vi "CPP_Aeroprobe-MultiProbeQuick.vi"() -> (5 "Plug in titles":string[](array[string]), 7 "Plug in values":string[](array[string]))   [LabVIEW 2013]
uses:
  Globals/Meas_global.vi
  Globals/Trav_pos_global.vi
panel:
  out "MultiProbeCals":string caption="DelimitedCalFileList (for MultiProbe)"
  in  "Calibration Folder Path":path=path "G:/5HoleProbe"
  in  "Old5HoleProbe?":bool
  in  "Mode":enum32{"Measure", "Take Zeroes"}(radio)=enum."Take Zeroes"
  in  "RunManually?":bool
  out "return type":i32
  out "p-p0":dbl[](array[numeric]) format="%#.5f"
  out "Temperature/C":dbl format="%#.1f"
  out "Pressure/mBar":dbl
  out "timeOfzero":timestamp
  out "zeroShift/mmH2O":dbl[](array[numeric]) format="%#.6f"
  out "Velocity":dbl
  out "W":dbl
  out "V":dbl
  out "U":dbl caption="u  m/s"
  # "!! 5-hole 1-5 must be connected to Channels 1-5 !!"
  # "Zero Info"
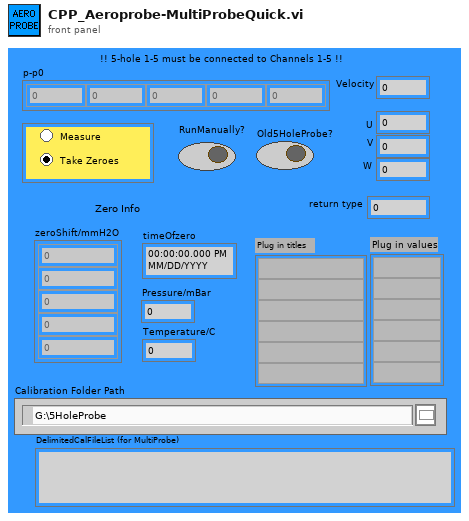
[diagram p1: front panel]
types:
  T1 = typedef "Post_Process.ctl" = enum16{"Take New Data", "Post Process Raw Data File"}
  T2 = typedef "Traverse_cluster.ctl" = cluster{"Start X":dbl, "Start Y":dbl, "Start Z":dbl, "End X":dbl, "End Y":dbl, "End Z":dbl, "No. of pts.":i32, "Spacing":T3, "Filename":path, "Tunnel Speed":dbl, "Averaging time (min)":dbl, "Extra Commands":string, "Specific Arguments":string, "Emission Rate (l/min)":dbl, "Trace Gas Concentration (%)":dbl, "Density Ratio":string, "Comments":string, "Row No":i32, "Row Type Selector":T4, "Completion time":string, "Row Duration (mins)":dbl, "No. of Valid pts.":i32, "Meas Setup File":string}
  T3 = typedef "Spacing.ctl" = enum16{"Linear", "Log", "Gauss", "Specified", "N/A"}
  T4 = typedef "Multi_run_mode.ctl" = enum16{"Move Traverse Only", "Set Tunnel Speed Only", "Set Source Only", "Set Measurement Conditions", "Single Measurement", "Vertical Profile", "Lateral Profile", "Longitudinal Profile", "Explore Volume", "Multi-Axis Profile", "Auto Calibrate", "Meas Fast FID Bkgnd", "Check Beam Power", "Scanning Valve Measurement", "Run VI Named:", "Set ADAM Ch", "Wait (minutes)", "Send Message", "Synchronize With:", "Fall Back to this Row", "Turn Off Row Repeating", "Blank Row", "Traverse 3D Volume"}
  T5 = typedef "Analysis_info_cluster.ctl" = cluster{"Colour":u32, "Inst type":T6, "Inst name":string, "Symbol":string, "Code name":string, "Extra Info":string, "Inst Array":T7, "Extra Titles":string[], "Extra Values":string[], "U":dbl, "u^2":dbl, "u^3":dbl, "u^4":dbl, "Skew_u":dbl, "Kurt_u":dbl, "Sd Error in Mean":dbl, "% u'/U":dbl, "X":dbl, "Y":dbl, "Z":dbl, "Timescale integral to 25%":dbl, "Sd Error in Variance":dbl, "Calib File":path, "Calib Constants":dbl[], "Output Position":bool, "Full Stats":bool, "Av Sampling Rate":dbl, "Av No of Samples":dbl, "Total Meas Time (s)":dbl, "ADAM Ch Name":string}
  T6 = typedef "Inst_type.ctl" = enum16{"Propeller anemometer", "Raw voltage", "Pressure Transducer", "Pitot-static tube", "Preston tube", "Hot wire", "Cross wire 1", "Cross wire 2", "Generic Linear", "Generic Polynomial", "Generic BackPoly", "Fast FID", "Thermocouple", "Cold wire", "Pulsed Wire", "LDA Vel", "LDA Tran time", "LDA Arr time"}
  T7 = typedef "Instrument_Array.ctl" = enum16{"PWA", "LDA", "Analogue"}
  T8 = cluster{"Analysis Info cluster[0]":T5, "Analysis Info cluster[1]":T5, "Analysis Info cluster[2]":T5, "Analysis Info cluster[3]":T5, "Analysis Info cluster[4]":T5, "Analysis Info cluster[5]":T5, "Analysis Info cluster[6]":T5}
  T9 = cluster{"Analysis Info cluster[0]":T5, "Analysis Info cluster[1]":T5, "Analysis Info cluster[2]":T5, "Analysis Info cluster[3]":T5, "Analysis Info cluster[4]":T5, "Analysis Info cluster[5]":T5, "Analysis Info cluster[6]":T5, "Analysis Info cluster[7]":T5, "Analysis Info cluster[8]":T5, "Analysis Info cluster[9]":T5, "Analysis Info cluster[10]":T5, "Analysis Info cluster[11]":T5, "Analysis Info cluster[12]":T5, "Analysis Info cluster[13]":T5}
  T10 = cluster{"[0]":dbl, "[1]":dbl, "[2]":dbl, "[3]":dbl, "[4]":dbl}
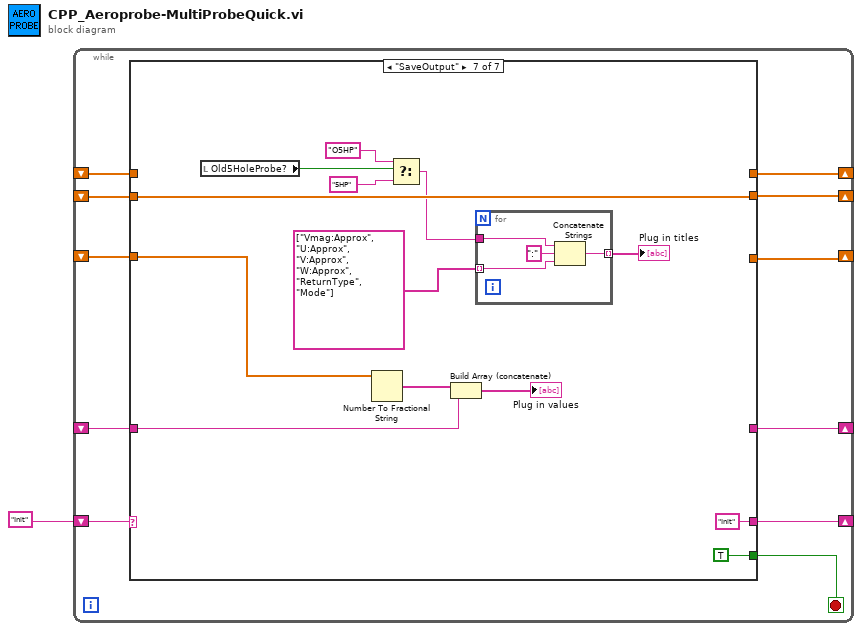
[diagram p0: block diagram]
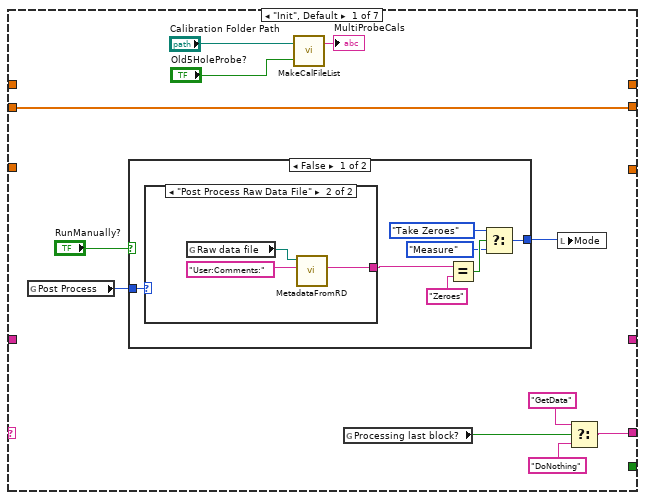
[diagram p2: hidden frame]
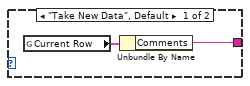
[diagram p3: hidden frame]
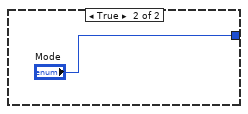
[diagram p4: hidden frame]
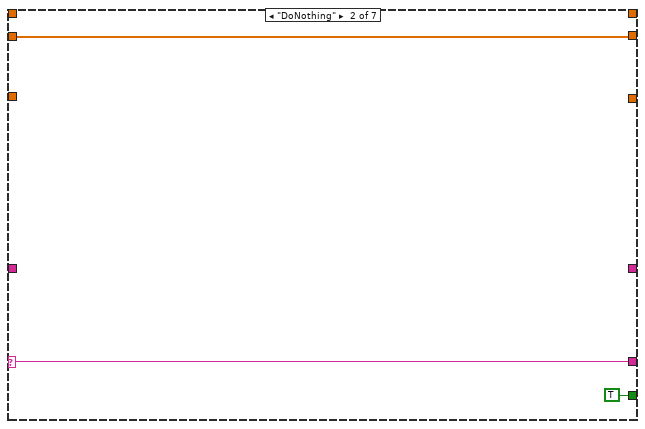
[diagram p5: hidden frame]
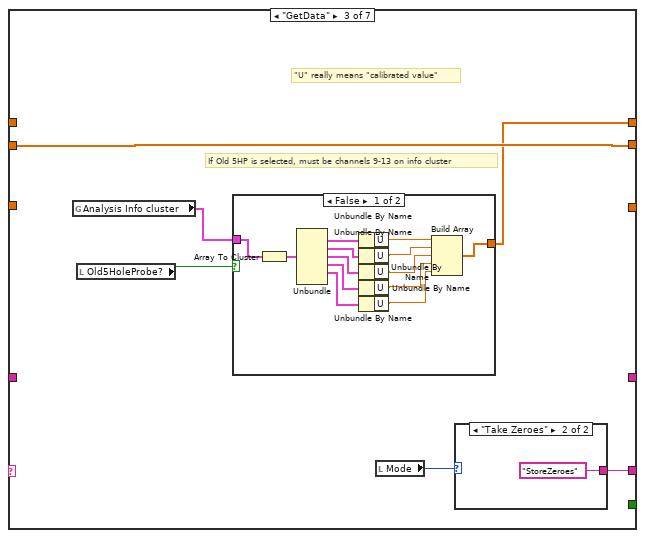
[diagram p6: hidden frame]
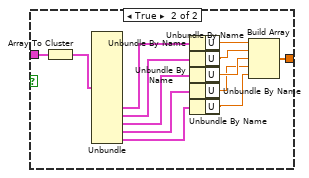
[diagram p7: hidden frame]
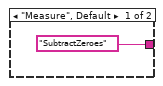
[diagram p8: hidden frame]
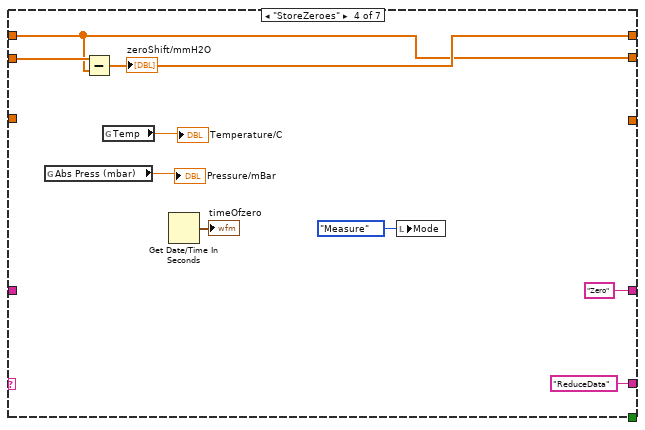
[diagram p9: hidden frame]
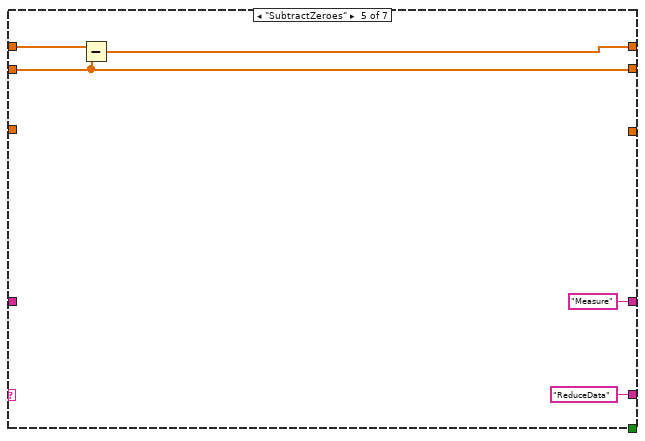
[diagram p10: hidden frame]
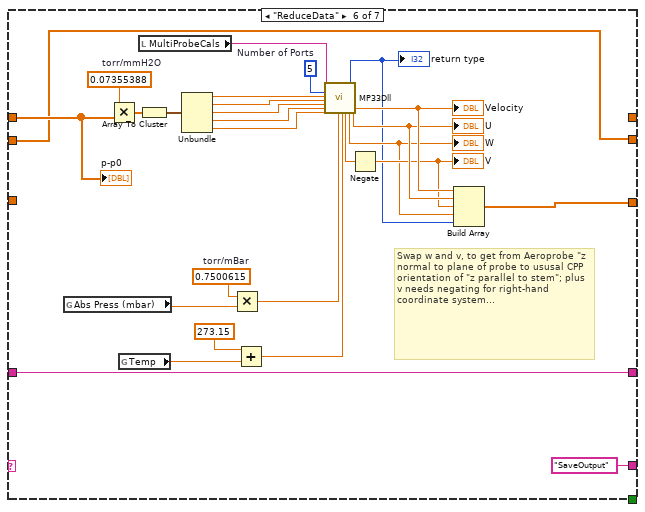
[diagram p11: hidden frame]
diagram:
  n1 = while {
    shift-right: [w11] -> _
    shift-left: "Init" -> [w12]
    shift-right: [w10] -> _
    shift-left: _ -> [w8]
    shift-right: [w9] -> _
    shift-left: _ -> [w7]
    shift-right: [w6] -> _
    shift-left: _ -> [w5]
    shift-right: [w3] -> _
    shift-left: _ -> [w2]
    stop <- w4 stop-if-true
    n2 = case shown="\"SaveOutput\"" w12 {
      selector: w12 -> [_ w39 _ _ _ _ _]
      tunnel: [w23 w39 w45 "ReduceData" "ReduceData" "SaveOutput" "Init"] -> w11
      tunnel: [_ _ w42 w80 w86 _ _] -> w10
      tunnel: [w19 w37 w44 w74 w85 w99 w127] -> w9
      tunnel: w8 -> [_ _ _ w74 w87 w108 _]
      tunnel: w7 -> [w19 w37 w44 w82 w85 w99 w127]
      tunnel: [_ _ _ _ _ w95 _] -> w6
      tunnel: w5 -> [_ _ _ _ _ _ w126]
      tunnel: [_ TRUE _ _ _ _ TRUE] -> w4
      tunnel: [_ _ _ "Zero" "Measure" w94 _] -> w3
      tunnel: w2 -> [_ _ _ _ _ w94 w121]
      frame "Init", Default {
        n3 = global read "Meas_global.vi" "Post Process"() -> (w16:T1)
        n4 = case shown="False" "RunManually?" {
          tunnel: [w30 "Mode"] -> w17
          tunnel: w16 -> [w24 _]
          frame False {
            n5 = case shown="\"Post Process Raw Data File\"" w24 {
              tunnel: [w31 w33] -> w29
              frame "Take New Data", Default {
                n6 = global read "Trav_pos_global.vi" "Current Row"() -> (w32:T2)
                n7 = Unbundle By Name(w32) -> ("Comments"=w31:string)
              }
              frame "Post Process Raw Data File" {
                n8 = global read "Meas_global.vi" "Raw data file"() -> (w35:path)
                n9 = call "MetadataFromRD.vi"("ChannelName"="User:Comments:", "Raw data file"=w35) -> ("ValueString"=w33:string)  [unwired: 8 in, 1 out]
              }
            }
            n10 = Equal?(x=w29, y="Zeroes") -> (x = y?=w27:bool)
            n11 = Select(t=enum32{"Measure", "Take Zeroes"}."Take Zeroes" ("Mode"), s=w27, f=enum32{"Measure", "Take Zeroes"}."Measure" ("Mode")) -> (s? t:f=w30:enum32{"Measure", "Take Zeroes"})
          }
          frame True {
          }
        }
        n12 = call "MakeCalFileList.vi"("Old5HoleProbe?"="Old5HoleProbe?", "Calibration Folder Path"="Calibration Folder Path") -> ("MultiProbeCals"=→"MultiProbeCals":string)  [unwired: 1 out]
        n13 = global read "Meas_global.vi" "Processing last block?"() -> (w22:bool)
        n14 = local write "Mode"(w17) -> ()
        n15 = Select(t="GetData", s=w22, f="DoNothing") -> (s? t:f=w23:string)
      }
      frame "DoNothing" {
      }
      frame "GetData" {
        # "If Old 5HP is selected, must be channels 9-13 on info cluster"
        # "\"U\" really means \"calibrated value\""
        n16 = global read "Meas_global.vi" "Analysis Info cluster"() -> (w43:T5[])
        n17 = local read "Old5HoleProbe?"() -> (w40:bool)
        n18 = case shown="False" w40 {
          tunnel: w43 -> [w47 w67]
          tunnel: [w46 w61] -> w42
          frame False {
            n19 = Array To Cluster(array=w47) -> (cluster=w53:T8)
            n20 = Unbundle(w53) -> ("Analysis Info cluster[1]"=w52:T5, "Analysis Info cluster[2]"=w51:T5, "Analysis Info cluster[3]"=w50:T5, "Analysis Info cluster[4]"=w49:T5, "Analysis Info cluster[5]"=w48:T5)  [unwired: 2 out]
            n21 = Unbundle By Name(w52) -> ("U"=w54:dbl)
            n22 = Unbundle By Name(w51) -> ("U"=w55:dbl)
            n23 = Unbundle By Name(w50) -> ("U"=w56:dbl)
            n24 = Unbundle By Name(w49) -> ("U"=w57:dbl)
            n25 = Unbundle By Name(w48) -> ("U"=w58:dbl)
            n26 = Build Array(w54, w55, w56, w57, w58) -> (w46:dbl[])
          }
          frame True {
            n27 = Array To Cluster(array=w67) -> (cluster=w68:T9)
            n28 = Unbundle(w68) -> ("Analysis Info cluster[9]"=w66:T5, "Analysis Info cluster[10]"=w65:T5, "Analysis Info cluster[11]"=w64:T5, "Analysis Info cluster[12]"=w63:T5, "Analysis Info cluster[13]"=w62:T5)  [unwired: 9 out]
            n29 = Unbundle By Name(w66) -> ("U"=w69:dbl)
            n30 = Unbundle By Name(w65) -> ("U"=w70:dbl)
            n31 = Unbundle By Name(w64) -> ("U"=w60:dbl)
            n32 = Unbundle By Name(w63) -> ("U"=w59:dbl)
            n33 = Unbundle By Name(w62) -> ("U"=w71:dbl)
            n34 = Build Array(w69, w70, w60, w59, w71) -> (w61:dbl[])
          }
        }
        n35 = local read "Mode"() -> (w41:enum32{"Measure", "Take Zeroes"})
        n36 = case shown="\"Take Zeroes\"" w41 {
          tunnel: ["SubtractZeroes" "StoreZeroes"] -> w45
          frame "Measure", Default {
          }
          frame "Take Zeroes" {
          }
        }
      }
      frame "StoreZeroes" {
        n37 = global read "Meas_global.vi" "Abs Press (mbar)"() -> (→"Pressure/mBar":dbl)
        n38 = Subtract(x=w82, y=w74) -> (x-y=w80:dbl[])
        "zeroShift/mmH2O" <- w80
        n39 = global read "Meas_global.vi" "Temp"() -> (→"Temperature/C":dbl)
        n40 = Get Date/Time In Seconds() -> (seconds since 1Jan1904=→"timeOfzero":timestamp)
        n41 = local write "Mode"(enum32{"Measure", "Take Zeroes"}."Measure" ("Mode")) -> ()
      }
      frame "SubtractZeroes" {
        n42 = Subtract(x=w87, y=w85) -> (x-y=w86:dbl[])
      }
      frame "ReduceData" {
        w109 = 0.07355388  # torr/mmH2O
        w113 = 0.7500615  # torr/mBar
        w110 = 5  # Number of Ports
        # "Swap w and v, to get from Aeroprobe \"z normal to plane of probe to ususal CPP orientation of \"z parallel to stem\"; plus v needs negating for right-hand coordinate system..."
        n43 = global read "Meas_global.vi" "Abs Press (mbar)"() -> (w90:dbl)
        n44 = Multiply(x=w109, y=w108) -> (x*y=w107:dbl[])
        n45 = global read "Meas_global.vi" "Temp"() -> (w91:dbl)
        n46 = local read "MultiProbeCals"() -> (w88:string)
        n47 = Array To Cluster(array=w107) -> (cluster=w106:T10)
        n48 = Unbundle(w106) -> ("[0]"=w105:dbl, "[1]"=w104:dbl, "[2]"=w103:dbl, "[3]"=w102:dbl, "[4]"=w101:dbl)
        n49 = Multiply(x=w113, y=w90) -> (x*y=w112:dbl)
        n50 = Add(x=273.15, y=w91) -> (x+y=w114:dbl)
        n51 = call "MP33Dll.vi"("MultiProbeCals"=w88, "Number of Ports"=w110, "P1 Torr"=w105, "P2 Torr"=w104, "P3 Torr"=w103, "P4 Torr"=w102, "P5 Torr"=w101, "Pref Torr"=w112, "TTot Kelvin"=w114) -> ("w m/s"=w96:dbl, "return type"=w89:i32, "v m/s"=w92:dbl, "VMagn m/s"=w98:dbl, "u  m/s"=w97:dbl)  [unwired: 8 in, 6 out]
        "U" <- w97
        "W" <- w92
        "Velocity" <- w98
        "return type" <- w89
        n52 = Negate(x=w96) -> (-x=w93:dbl)
        "V" <- w93
        n53 = Build Array(w98, w97, w93, w92, w89) -> (w95:dbl[])
        "p-p0" <- w108
      }
      frame "SaveOutput" {
        n54 = local read "Old5HoleProbe?"() -> (w119:bool)
        n55 = Number To Fractional String(number=w126) -> (F-format string=w125:string[])  [unwired: 3 in]
        n56 = Select(t="O5HP", s=w119, f="5HP") -> (s? t:f=w116:string)
        n57 = Build Array (concatenate)(w125, w121) -> (→"Plug in values":string[])
        n58 = for {
          tunnel: string[] ["Vmag:Approx", "U:Approx", "V:Approx", "W:Approx", "ReturnType", "Mode"] ("Plug in titles") -> [w129] mode=indexing
          tunnel: w116 -> [w131]
          tunnel: [w128] -> w115 mode=indexing
          n59 = Concatenate Strings(w131, ":" ("string"), w129) -> (w128:string)
        }
        "Plug in titles" <- w115
      }
    }
  }
